vi "Build New AIM ARINC 429 Custom Device.vi"(7 "Base System Definition File":path=path "Support/Base.nivssdf", 11 "Output System Definition File":path=path "Support/Scripted AIM ARINC 429.nivssdf") -> (3 "AIM ARINC 429 System Definition":path)   [LabVIEW 2024]
doc: "Overview: Demonstrates using the Ballard ARINC 429 scripting API to configure the custom device by building from configuration clusters. \n\nInstructions:\n1. Specify the Hardware Configuration File. The hardware configuration file must be consistent with the schema installed by the Ballard hardware driver at C:\\Program Files (x86)\\Astronics Ballard Technology LabVIEW Driver\\Help\\index.html. The hardware configuration file must also be consistent with the configuration in this example VI.\n2. (VeriStand) Optionally, you may open the Output System Definition File in VeriStand, configure the Target, and deploy the scripted system definition to perform avionics bus communications with Ballard ARINC 429 hardware."
uses:
  <vilib>/addons/VeriStand Custom Device Scripting APIs/AIM ARINC 429/Shared/Direction.ctl
  <vilib>/addons/VeriStand Custom Device Scripting APIs/AIM ARINC 429/Shared/SDI.ctl
  <vilib>/addons/VeriStand Custom Device Scripting APIs/AIM ARINC 429/Shared/Transfer Type.ctl
  <vilib>/addons/VeriStand Custom Device Scripting APIs/AIM ARINC 429/Shared/Parameter Definition.ctl
  <vilib>/NI/NI VeriStand Encoding and Decoding/Encoding.ctl
  <vilib>/addons/VeriStand Custom Device Scripting APIs/AIM ARINC 429/Shared/Device Parameters.ctl
  <vilib>/addons/VeriStand Custom Device Scripting APIs/AIM ARINC 429/Shared/Transfer Speed.ctl
  NationalInstruments.VeriStand.SystemDefinitionAPI
  AIM ARINC 429 Scripting Examples.lvlib
  <vilib>/addons/VeriStand Custom Device Scripting APIs/AIM ARINC 429/Shared/AIM ARINC 429 Shared.lvlib
  <vilib>/NI/NI VeriStand Encoding and Decoding/Encoding and Decoding.lvlib
  <vilib>/addons/VeriStand Custom Device Scripting APIs/AIM ARINC 429/Scripting/AIM/AIM ARINC 429 Scripting.lvlib
panel:
  # "Overview: Demonstrates using the AIM ARINC 429 scripting API to configure the custom device by building from configuration clusters. \n\nInstructions:\n1. Run this example VI, which will create an instance of the AIM ARINC 429 Custom Deivce in a VeriStand system definition with a configuration matching the constants on the block diagram.\n2. (VeriStand) Optionally, you may open the Output System Definition File in VeriStand, configure the Target, and deploy the scripted system definition to perform avionics bus communications with AIM ARINC 429 hardware."
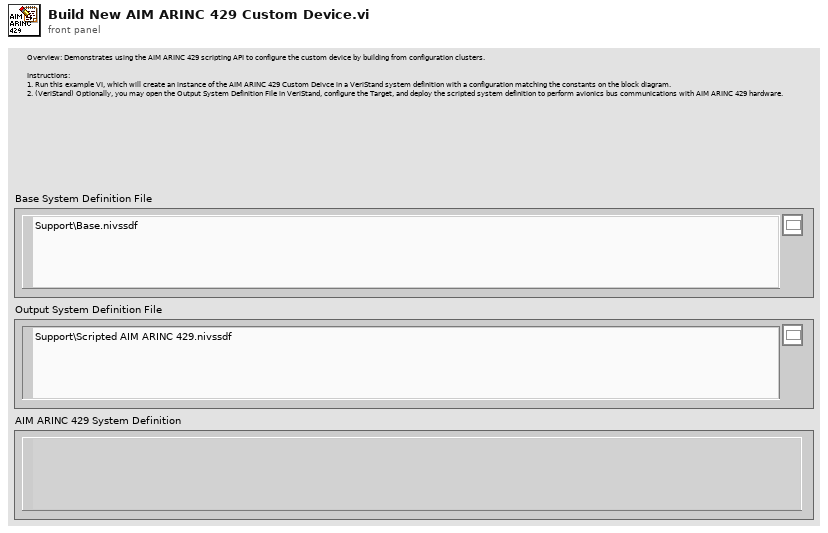
[diagram p1: front panel]
types:
  T1 = typedef "AIM ARINC 429 Shared.lvlib/Transfer Speed.ctl" = enum16{"LO (12.5 kb/s)", "HI (100 kb/s)"}
  T2 = typedef "AIM ARINC 429 Shared.lvlib/Device Parameters.ctl" = cluster{"pxi slot":u8, "coupling mode":u32}
  T3 = typedef "AIM ARINC 429 Shared.lvlib/Parameter Definition.ctl" = cluster{"start index":i32, "size":i32, "encoding":T4, "signed":bool, "scale multiplier":dbl, "scale offset":dbl, "default value":dbl}
  T4 = typedef "Encoding and Decoding.lvlib/Encoding.ctl" = enum16{"BNR", "BCD", "Discrete"}
  T5 = typedef "AIM ARINC 429 Shared.lvlib/Direction.ctl" = enum16{"Rx", "Tx"}
  T6 = typedef "AIM ARINC 429 Shared.lvlib/Transfer Type.ctl" = enum16{"Scheduled", "Acyclic", "Block", "Strobe"}
  T7 = typedef "AIM ARINC 429 Shared.lvlib/SDI.ctl" = i32
  T8 = typedef "Custom Device API.lvlib/Custom Device Item Ref.ctl" = u64
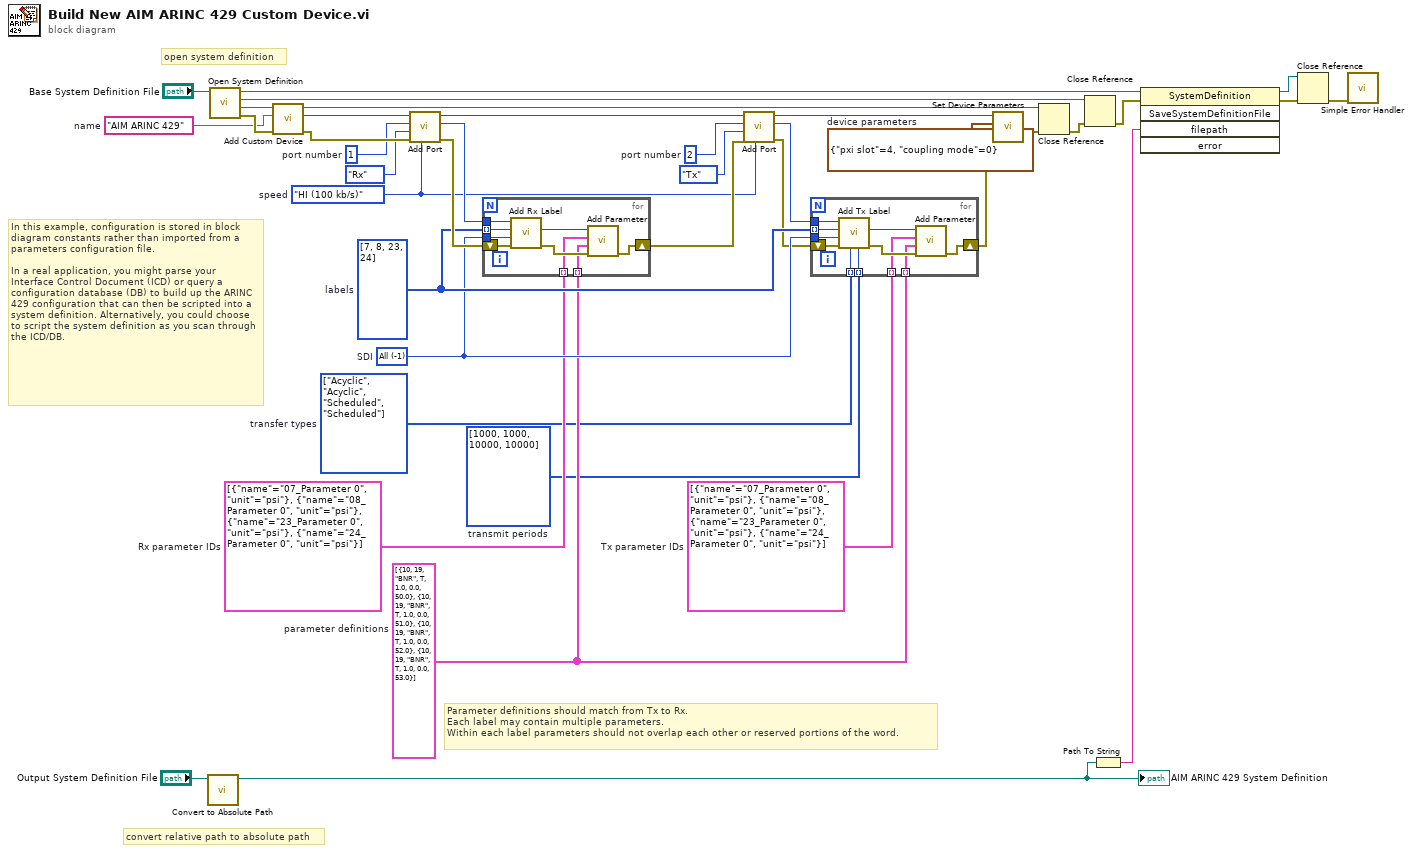
[diagram p0: block diagram]
diagram:
  w1 = u32[] [1000, 1000, 10000, 10000]  # transmit periods
  w2 = Transfer_Speed."HI (100 kb/s)"  # speed
  w3 = T2 {"pxi slot"=4, "coupling mode"=0}  # device parameters
  w8 = cluster{"name":string, "unit":string}[] [{"name"="07_Parameter 0", "unit"="psi"}, {"name"="08_Parameter 0", "unit"="psi"}, {"name"="23_Parameter 0", "unit"="psi"}, {"name"="24_Parameter 0", "unit"="psi"}]  # Tx parameter IDs
  w10 = T3[] [{"start index"=10, "size"=19, "encoding"=enum."BNR", "signed"=TRUE, "scale multiplier"=1.0, "scale offset"=0.0, "default value"=50.0}, {"start index"=10, "size"=19, "encoding"=enum."BNR", "signed"=TRUE, "scale multiplier"=1.0, "scale offset"=0.0, "default value"=51.0}, {"start index"=10, "size"=19, "encoding"=enum."BNR", "signed"=TRUE, "scale multiplier"=1.0, "scale offset"=0.0, "default value"=52.0}, {"start index"=10, "size"=19, "encoding"=enum."BNR", "signed"=TRUE, "scale multiplier"=1.0, "scale offset"=0.0, "default value"=53.0}]  # parameter definitions
  w11 = cluster{"name":string, "unit":string}[] [{"name"="07_Parameter 0", "unit"="psi"}, {"name"="08_Parameter 0", "unit"="psi"}, {"name"="23_Parameter 0", "unit"="psi"}, {"name"="24_Parameter 0", "unit"="psi"}]  # Rx parameter IDs
  w19 = u16 2  # port number
  w9 = T6[] [enum."Acyclic", enum."Acyclic", enum."Scheduled", enum."Scheduled"] items=["Scheduled", "Acyclic", "Block", "Strobe"]  # transfer types
  w13 = T7 -1 items=["All"=-1, "0 (b00)"=0, "1 (b01)"=1, "2 (b10)"=2, "3 (b11)"=3]  # SDI
  w14 = u32[] [7, 8, 23, 24]  # labels
  w21 = u16 1  # port number
  w26 = "AIM ARINC 429"  # name
  # "open system definition"
  # "convert relative path to absolute path"
  # "Parameter definitions should match from Tx to Rx.\nEach label may contain multiple parameters.\nWithin each label parameters should not overlap each other or reserved portions of the word."
  # "In this example, configuration is stored in block diagram constants rather than imported from a parameters configuration file.\n\nIn a real application, you might parse your Interface Control Document (ICD) or query a configuration database (DB) to build up the ARINC 429 configuration that can then be scripted into a system definition. Alternatively, you could choose to script the system definition as you scan through the ICD/DB."
  # "8."
  n1 = call "Convert to Absolute Path.vi"("system definition file"="Output System Definition File") -> ("absolute path"=w7:path)  [unwired: 10 in]
  "AIM ARINC 429 System Definition" <- w7
  n2 = call "Open System Definition.vi"("system definition file"="Base System Definition File") -> ("error out"=w29:errorcluster, "target"=w28:refnum<k24>, "root"=w31:refnum<k24>, "system definition"=w32:refnum<k24>)  [unwired: 7 in]
  n3 = call <vilib>:"Add Custom Device.vi"("error in"=w29, "name"=w26, "target"=w28) -> ("error out"=w24:errorcluster, "AIM ARINC 429 custom device"=w25:T8, "target out"=w27:refnum<k24>)  [unwired: 6 in]
  n4 = call <vilib>:"Add Port.vi"("speed"=w2, "error in"=w24, "direction"=Direction."Rx", "port number"=w21, "custom device ref"=w25) -> ("error out"=w22:errorcluster, "port"=w23:T8, "custom device ref out"=w17:T8)  [unwired: 4 in]
  n5 = for {
    tunnel: w23 -> [w48]
    tunnel: w13 -> [w46]
    shift-right: [w42] -> w16
    shift-left: w22 -> [w47]
    tunnel: w14 -> [w43] mode=indexing
    tunnel: w11 -> [w41] mode=indexing
    tunnel: w10 -> [w40] mode=indexing
    n6 = call <vilib>:"Add Rx Label.vi"("error in"=w47, "SDI value"=w46, "label value"=w43, "port ref"=w48) -> ("error out"=w44:errorcluster, "label"=w45:T8)  [unwired: 5 in, 1 out]
    n7 = call <vilib>:"Add Parameter.vi"("error in"=w44, "parameter encoding"=w40, "parameter definition"=w41, "label ref"=w45) -> ("error out"=w42:errorcluster)  [unwired: 5 in, 2 out]
  }
  n8 = call <vilib>:"Add Port.vi"("speed"=w2, "error in"=w16, "direction"=Direction."Tx", "port number"=w19, "custom device ref"=w17) -> ("error out"=w12:errorcluster, "port"=w15:T8, "custom device ref out"=w6:T8)  [unwired: 4 in]
  n9 = for {
    tunnel: w15 -> [w59]
    tunnel: w13 -> [w57]
    shift-right: [w53] -> w5
    shift-left: w12 -> [w58]
    tunnel: w14 -> [w54] mode=indexing
    tunnel: w8 -> [w52] mode=indexing
    tunnel: w10 -> [w51] mode=indexing
    tunnel: w9 -> [w50] mode=indexing
    tunnel: w1 -> [w49] mode=indexing
    n10 = call <vilib>:"Add Tx Label.vi"("scheduled transmit period (us)"=w49, "transfer type"=w50, "error in"=w58, "SDI value"=w57, "label value"=w54, "port ref"=w59) -> ("error out"=w55:errorcluster, "label"=w56:T8)  [unwired: 3 in, 1 out]
    n11 = call <vilib>:"Add Parameter.vi"("error in"=w55, "parameter encoding"=w51, "parameter definition"=w52, "label ref"=w56) -> ("error out"=w53:errorcluster)  [unwired: 5 in, 2 out]
  }
  n12 = call <vilib>:"Set Device Parameters.vi"("error in"=w5, "device parameters"=w3, "custom device"=w6) -> ("error out"=w4:errorcluster)  [unwired: 7 in, 1 out]
  n13 = Close Reference(reference=w27, error in (no error)=w4) -> (error out=w30:errorcluster)
  n14 = Close Reference(reference=w31, error in (no error)=w30) -> (error out=w35:errorcluster)
  n15 = Path To String(path=w7) -> (string=w38:string)
  n16 = invoke class="SystemDefinition" method="SaveSystemDefinitionFile"(reference=w32, error in=w35, "filepath"=w38) -> (reference out=w36:refnum<k24>, error out=w37:errorcluster)  [unwired: 2 in, 3 out]
  n17 = Close Reference(reference=w36, error in (no error)=w37) -> (error out=w34:errorcluster)
  n18 = call <vilib>:"Simple Error Handler.vi"("error in (no error)"=w34) -> ()  [unwired: 1 in, 8 out]
